vi "SDG60Initialize.vi"(2 "error in (no error)":errorcluster, 3 "VISA resource name":refnum<visa-resource-name>="USB0::0xF4EC::0x1101::SDG6XEBC5R0119::INSTR") -> (0 "error out":errorcluster, 1 "VISA resource name out":refnum<visa-resource-name>)   [LabVIEW 2018]
doc: "Establishes communication with the instrument and optionally performs an instrument identification query and/or an instrument reset. It also places the instrument in a default state needed for other instrument driver operations. Therefore, call this VI before calling other instrument driver VIs for this instrument. Generally, you need to call the Initialize VI only once at the beginning of an application."
panel:
  # "Will reset to default settings. \nThis has 4Vpp 1kHz \nsine wave"
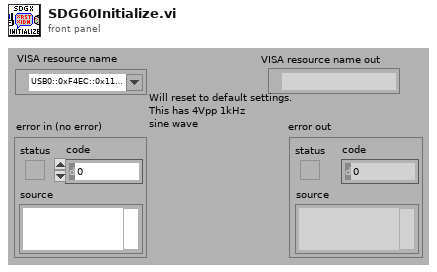
[diagram p1: front panel]
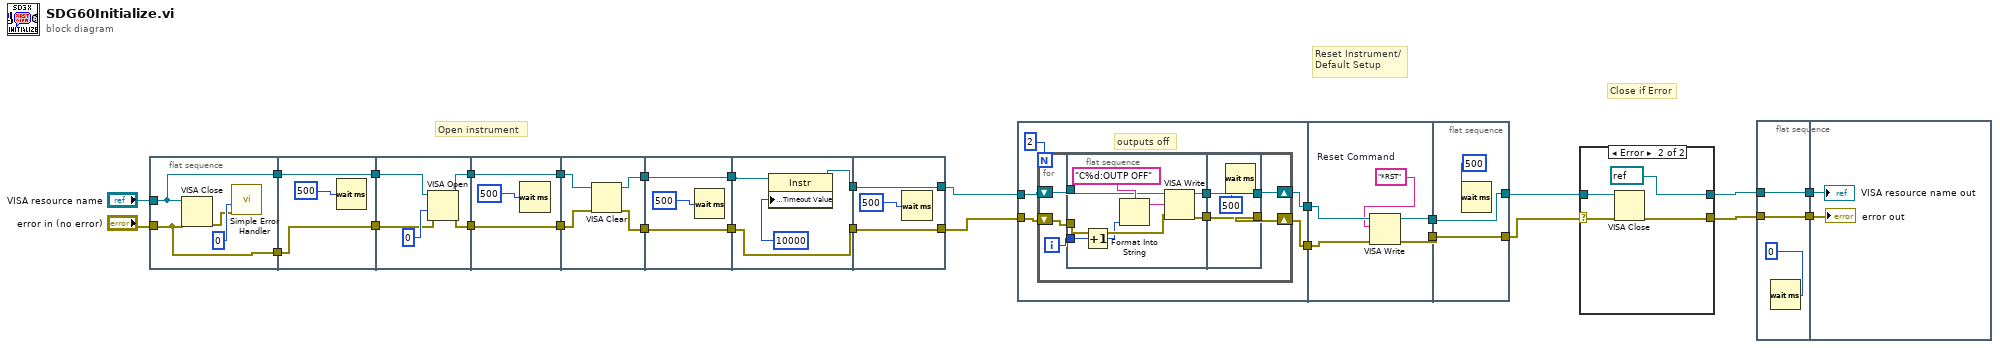
[diagram p0: block diagram]
diagram:
  # "Close if Error"
  # "Reset Instrument/\nDefault Setup"
  # "Open instrument"
  n1 = flat-sequence {
    tunnel: "error in (no error)" -> [w30]
    tunnel: "VISA resource name" -> [w29]
    tunnel: [w30] -> w22
    tunnel: [w29] -> w21
    tunnel: w22 -> [w34]
    tunnel: w21 -> [w33]
    tunnel: [w34] -> w20
    tunnel: [w33] -> w19
    tunnel: w20 -> [w38]
    tunnel: w19 -> [w39]
    tunnel: [w37] -> w18
    tunnel: [w36] -> w17
    tunnel: w18 -> [w43]
    tunnel: w17 -> [w42]
    tunnel: [w43] -> w16
    tunnel: [w42] -> w15
    tunnel: w16 -> [w46]
    tunnel: w15 -> [w47]
    tunnel: [w45] -> w14
    tunnel: [w44] -> w13
    tunnel: w14 -> [w50]
    tunnel: w13 -> [w49]
    tunnel: [w50] -> w12
    tunnel: [w49] -> w11
    tunnel: w12 -> [w53]
    tunnel: w11 -> [w52]
    tunnel: [w52] -> w10
    tunnel: [w51] -> w9
    tunnel: [w56] -> w8
    tunnel: [w57] -> w7
    tunnel: w10 -> [w57]
    tunnel: w9 -> [w56]
    frame #0 {
      n2 = VISA Close(VISA resource name=w29, error in (no error)=w30) -> (error out=w31:errorcluster)
      n3 = call <vilib>:"Simple Error Handler.vi"("type of dialog (OK msg:1)"=0, "error in (no error)"=w31) -> ()  [unwired: 3 in, 5 out]
    }
    frame #1 {
      n4 = Wait (ms)(milliseconds to wait=500) -> ()  [unwired: 1 out]
    }
    frame #2 {
      n5 = VISA Open(access mode=u32 0, error in (no error)=w38, VISA resource name=w39) -> (VISA resource name=w36:refnum<visa-resource-name>, error out=w37:errorcluster)  [unwired: 2 in]
    }
    frame #3 {
      n6 = Wait (ms)(milliseconds to wait=500) -> ()  [unwired: 1 out]
    }
    frame #4 {
      n7 = VISA Clear(VISA resource name=w47, error in (no error)=w46) -> (VISA resource name out=w45:refnum<visa-resource-name>, error out=w44:errorcluster)
    }
    frame #5 {
      n8 = Wait (ms)(milliseconds to wait=500) -> ()  [unwired: 1 out]
    }
    frame #6 {
      n9 = property class="Instr"(reference=w53, "General Settings:Timeout Value"=u32 10000) -> (reference out=w51:refnum<visa-resource-name>)  [unwired: 1 in, 1 out]
    }
    frame #7 {
      n10 = Wait (ms)(milliseconds to wait=500) -> ()  [unwired: 1 out]
    }
  }
  n11 = flat-sequence {
    tunnel: w8 -> [w61]
    tunnel: w7 -> [w59]
    tunnel: [w60] -> w4
    tunnel: [w58] -> w3
    tunnel: w4 -> [w85]
    tunnel: w3 -> [w81]
    tunnel: [w84] -> w6
    tunnel: [w83] -> w5
    tunnel: [w87] -> w27
    tunnel: [w88] -> w28
    tunnel: w6 -> [w88]
    tunnel: w5 -> [w87]
    frame #0 {
      # "outputs off"
      n12 = for {
        N: 2 -> [_]
        shift-right: [w67] -> w60
        shift-left: w61 -> [w68]
        shift-right: [w66] -> w58
        shift-left: w59 -> [w65]
        i -> [w69]
        n13 = flat-sequence {
          tunnel: w69 -> [w70]
          tunnel: w68 -> [w75]
          tunnel: w65 -> [w72]
          tunnel: [w74] -> w64
          tunnel: [w73] -> w63
          tunnel: [w79] -> w66
          tunnel: [w80] -> w67
          tunnel: w64 -> [w80]
          tunnel: w63 -> [w79]
          frame #0 {
            n14 = Increment(x=w70) -> (x+1=w71:i32)
            n15 = Format Into String(format string="C%d:OUTP OFF", w71) -> (resulting string=w76:string)  [unwired: 2 in, 1 out]
            n16 = VISA Write(VISA resource name=w75, write buffer=w76, error in (no error)=w72) -> (VISA resource name out=w74:refnum<visa-resource-name>, error out=w73:errorcluster)  [unwired: 1 out]
          }
          frame #1 {
            n17 = Wait (ms)(milliseconds to wait=500) -> ()  [unwired: 1 out]
          }
        }
      }
    }
    frame #1 {
      w82 = "*RST"  # Reset Command
      n18 = VISA Write(VISA resource name=w85, write buffer=w82, error in (no error)=w81) -> (VISA resource name out=w84:refnum<visa-resource-name>, error out=w83:errorcluster)  [unwired: 1 out]
    }
    frame #2 {
      n19 = Wait (ms)(milliseconds to wait=500) -> ()  [unwired: 1 out]
    }
  }
  n20 = case shown="Error" w27 {
    selector: w27 -> [w89 w92]
    tunnel: w28 -> [w90 w93]
    tunnel: [w90 refnum<visa-resource-name> refnum ("VISA resource name out")] -> w26
    tunnel: [w89 w91] -> w25
    frame No Error {
    }
    frame Error {
      n21 = VISA Close(VISA resource name=w93, error in (no error)=w92) -> (error out=w91:errorcluster)
    }
  }
  n22 = flat-sequence {
    tunnel: [w97] -> w2
    tunnel: [w96] -> w1
    tunnel: w26 -> [w97]
    tunnel: w25 -> [w96]
    tunnel: w2 -> [w99]
    tunnel: w1 -> [w98]
    frame #0 {
      n23 = Wait (ms)(milliseconds to wait=0) -> ()  [unwired: 1 out]
    }
    frame #1 {
      "VISA resource name out" <- w99
      "error out" <- w98
    }
  }
